vi "Is Closed.vi"(11 "Event in":refnum<class "Event.lvclass">) -> (2 "Is Closed?":bool)   [LabVIEW 2022 SP3, in "Enclave.lvlib" / "Event.lvclass"]
uses:
  Event.lvclass
  Event.lvclass/Event.ctl
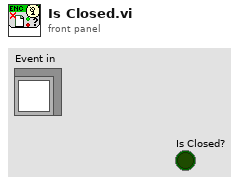
[diagram p1: front panel]
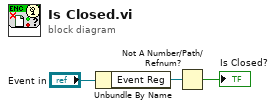
[diagram p0: block diagram]
diagram:
  n1 = Unbundle By Name("Event in") -> ("Event Reg"=w2:refnum<event-registration>)
  n2 = Not A Number/Path/Refnum?(number/path/refnum=w2) -> (NaN/Path/Refnum?=→"Is Closed?":bool)
